vi "Compile Status Channels.vi"(8 "error in (no error)":errorcluster, 10 "Channel Descriptors in":T1, 11 "Custom Device Ref":T8 format="%.0x") -> (0 "error out":errorcluster, 2 "Channel Descriptors out":T1, 3 "Custom Device Ref dup":T8 format="%.0x")   [LabVIEW 2011, in "Engine Sim System Explorer.lvlib"]
uses:
  Engine Sim System Explorer.lvlib
  <vilib>/NI Veristand/Custom Device API/Custom Device Item Ref.ctl
  Shared/Channel Descriptors.ctl
  Shared/FPGA Write Descriptor.ctl
  Shared/InputChannelTypes.ctl
  <vilib>/rvi/DataTransferAndStorage/Container/Common/niFpgaDataTypeControl.ctl
  Shared/FPGA Read Descriptor.ctl
  Shared/OutputChannelTypes.ctl
  Shared/Status Chan Descriptor.ctl
  Shared/Engine Simulation Global.vi
  <vilib>/NI Veristand/Custom Device Tools/Custom Device Utility Library/NI VeriStand - Search for Item by GUID.vi
  <vilib>/NI Veristand/Custom Device Tools/Custom Device Utility Library/NI VeriStand - Search for Item by Name.vi
  <vilib>/NI Veristand/Custom Device Tools/Custom Device Utility Library/Custom Device Utility Library.lvlib
  Engine Simulation Shared.lvlib
  <vilib>/NI Veristand/Custom Device API/Custom Device API.lvlib
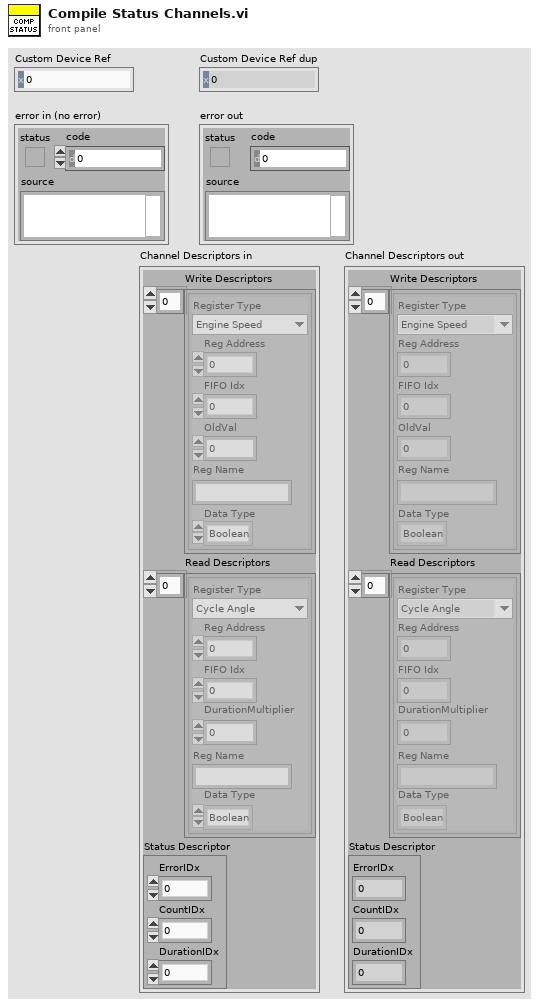
[diagram p1: front panel]
types:
  T1 = typedef "Engine Simulation Shared.lvlib/Channel Descriptors.ctl" = cluster{"Write Descriptors":T2[], "Read Descriptors":T5[], "Status Descriptor":T7}
  T2 = typedef "Engine Simulation Shared.lvlib/FPGA Write Descriptor.ctl" = cluster{"Register Type":T3, "Reg Address":u32, "FIFO Idx":i32, "OldVal":dbl, "Reg Name":string, "Data Type":T4}
  T3 = typedef "Engine Simulation Shared.lvlib/InputChannelTypes.ctl" = enum16{"Engine Speed", "Offset"}
  T4 = typedef "niFpgaDataTypeControl.ctl" = enum32{"Boolean", "I8", "I16", "I32", "I64", "U8", "U16", "U32", "U64", "FXP", "CustomControl"}
  T5 = typedef "Engine Simulation Shared.lvlib/FPGA Read Descriptor.ctl" = cluster{"Register Type":T6, "Reg Address":u32, "FIFO Idx":i32, "DurationMultiplier":dbl, "Reg Name":string, "Data Type":T4}
  T6 = typedef "Engine Simulation Shared.lvlib/OutputChannelTypes.ctl" = enum16{"Cycle Angle", "Crank Angle", "Time Duration", "Angle Duration", "Start Angle", "End Angle"}
  T7 = typedef "Engine Simulation Shared.lvlib/Status Chan Descriptor.ctl" = cluster{"ErrorIDx":i32, "CountIDx":i32, "DurationIDx":i32}
  T8 = typedef "Custom Device API.lvlib/Custom Device Item Ref.ctl" = u64
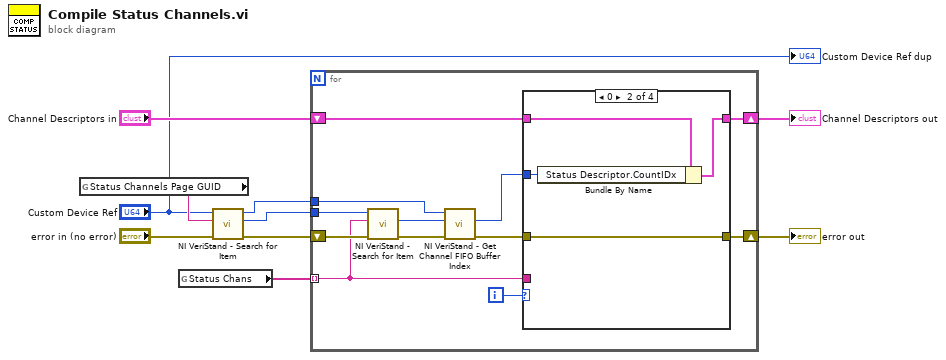
[diagram p0: block diagram]
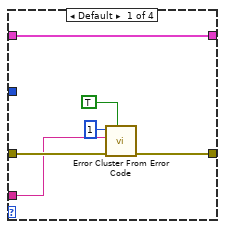
[diagram p2: hidden frame]
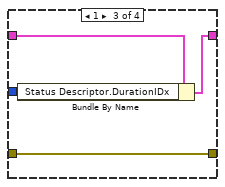
[diagram p3: hidden frame]
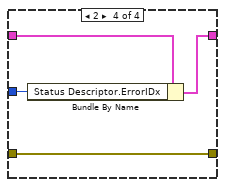
[diagram p4: hidden frame]
diagram:
  n1 = global read "Engine Simulation Global.vi" "Status Channels Page GUID"() -> (w9:string)
  n2 = global read "Engine Simulation Global.vi" "Status Chans"() -> (w6:string[])
  n3 = call-poly <vilib>:"NI VeriStand - Search for Item.vi"("error in"="error in (no error)", "Item GUID"=w9, "Section Ref in"="Custom Device Ref") -> ("error out"=w8:errorcluster, "Item Ref"=w7:T8, "Section Ref out"=w4:T8)  [unwired: 5 in, 1 out]
  n4 = for {
    tunnel: w7 -> [w21]
    shift-right: [w14] -> w2
    shift-left: w8 -> [w22]
    tunnel: w6 -> [w13] mode=indexing
    tunnel: w4 -> [w16]
    shift-right: [w11] -> w3
    shift-left: "Channel Descriptors in" -> [w12]
    i -> [w20]
    n5 = call-poly <vilib>:"NI VeriStand - Search for Item.vi"("error in"=w22, "Item Name"=w13, "Section Ref in"=w21) -> ("error out"=w19:errorcluster, "Item Ref"=w17:T8)  [unwired: 5 in, 2 out]
    n6 = call <vilib>:"NI VeriStand - Get Channel FIFO Buffer Index.vi"("error in"=w19, "Channel Ref"=w17, "Device Ref in"=w16) -> ("error out"=w18:errorcluster, "Channel FIFO Buffer Index"=w15:i32)  [unwired: 4 in, 3 out]
    n7 = case shown="0" w20 {
      tunnel: w18 -> [w28 w31 w35 w39]
      tunnel: w15 -> [_ w32 w36 w40]
      tunnel: [w27 w31 w35 w39] -> w14
      tunnel: [w23 w30 w34 w38] -> w11
      tunnel: w13 -> [w25 _ _ _]
      tunnel: w12 -> [w23 w29 w33 w37]
      frame Default {
        n8 = call <vilib>:"Error Cluster From Error Code.vi"("show call chain? (False)"=TRUE, "error in (no error)"=w28, "error message (\"\")"=w25, "error code (0)"=1) -> ("error out"=w27:errorcluster)  [unwired: 5 in]
      }
      frame 0 {
        n9 = Bundle By Name(cluster=w29, "Status Descriptor.CountIDx"=w32) -> (w30:T1)
      }
      frame 1 {
        n10 = Bundle By Name(cluster=w33, "Status Descriptor.DurationIDx"=w36) -> (w34:T1)
      }
      frame 2 {
        n11 = Bundle By Name(cluster=w37, "Status Descriptor.ErrorIDx"=w40) -> (w38:T1)
      }
    }
  }
  "error out" <- w2
  "Channel Descriptors out" <- w3
  "Custom Device Ref dup" <- "Custom Device Ref"
